vi "xiCam - Create.vi"(8 "error in (no error)":errorcluster) -> (0 "error out":errorcluster, 3 "new xiCam":refnum<k24>)   [LabVIEW 2015]
doc: "Creates a xiCam object."
uses:
  C:/GIT/Cameras3.x/Integrations/Labview/xiLib/xiLIB_32bit/xiLIB/xiCamLib/API/x86/xiApi.NET.dll
  xiLIB_32bit/xiLIB/xiCamLib/API/x86/xiApi.NET.dll
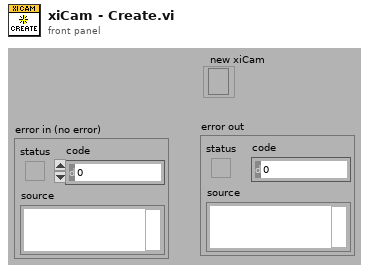
[diagram p1: front panel]
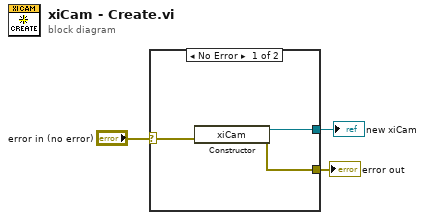
[diagram p0: block diagram]
diagram:
  n1 = case shown="No Error" "error in (no error)" {
    selector: "error in (no error)" -> [w5 _]
    tunnel: [w6 _] -> w3
    tunnel: [w4 _] -> w1
    frame No Error {
      n2 = constructor class="xiCam"(error in=w5) -> (reference out=w6:refnum<k24>, error out=w4:errorcluster)  [unwired: 2 in, 1 out]
    }
    frame Error {
    }
  }
  "new xiCam" <- w3
  "error out" <- w1
